vi "Write_Template.vi"(8 "error in (no error)":errorcluster, 10 "Control In":cluster{"Numeric":dbl, "String":string}[](array[cluster]), 11 "Class in":refnum<class "dsfsdfsd.lvclass">) -> (0 "error out":errorcluster, 3 "Class out":refnum<class "dsfsdfsd.lvclass">)   [LabVIEW 2013]
uses:
  TestProject/Class1/dsfsdfsd.lvclass
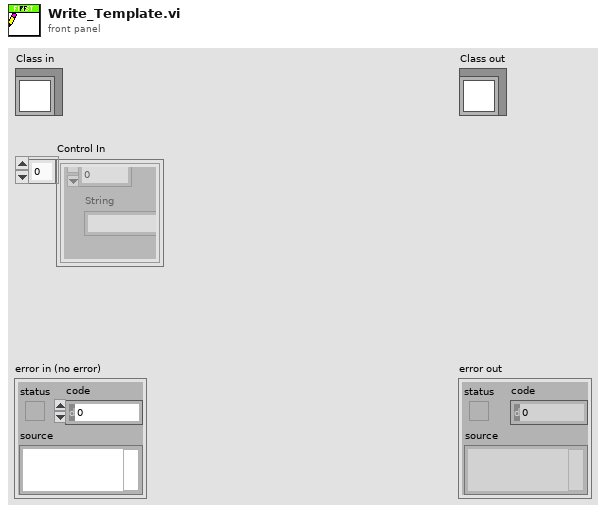
[diagram p1: front panel]
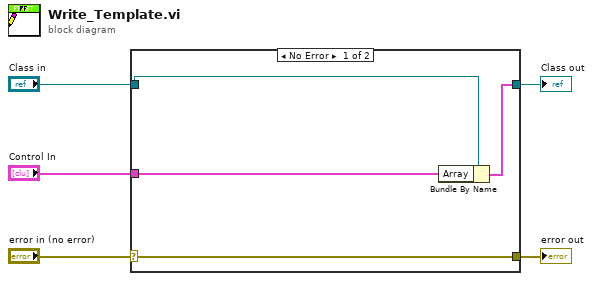
[diagram p0: block diagram]
diagram:
  n1 = case shown="No Error" "error in (no error)" {
    selector: "error in (no error)" -> [w9 w10]
    tunnel: [w9 w10] -> w4
    tunnel: [w7 w11] -> w2
    tunnel: "Class in" -> [w8 w11]
    tunnel: "Control In" -> [w6 _]
    frame No Error {
      n2 = Bundle By Name(cluster=w8, "Array"=w6) -> (w7:cluster{})
    }
    frame Error {
    }
  }
  "error out" <- w4
  "Class out" <- w2
